vi "Init.vi"() -> (3 "TEMPLATE Msg out":refnum<class "TEMPLATE Msg.lvclass">)   [LabVIEW 2020, in "_Template.lvlib" / "Templates.lvlib" / "TEMPLATE Msg.lvlib" / "TEMPLATE Msg.lvclass"]
uses:
  TEMPLATE Msg.lvclass
  jettl/jettl/Sender/Sender/Sender.lvclass
  TEMPLATE Msg.lvclass/TEMPLATE Msg.ctl
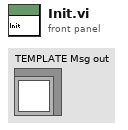
[diagram p1: front panel]
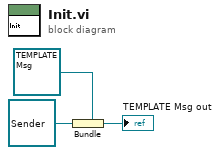
[diagram p0: block diagram]
diagram:
  n1 = Bundle "Bundle"(cluster=refnum<class "TEMPLATE Msg.lvclass"> refnum ("TEMPLATE Msg Strategy out"), refnum<class "Sender.lvclass"> refnum ("Sender")) -> (→"TEMPLATE Msg out":refnum<class "TEMPLATE Msg.lvclass">)
